vi "Write ITX.vi"(6 "Commands":string, 8 "error in":errorcluster, 9 "Notes":string, 10 "Data (Dictionary)":T1[](array[typedef]), 11 "filename":path) -> (0 "error out":errorcluster, 3 "file":path)   [LabVIEW 2019, in "LV-Data.ITX.lvclass"]
uses:
  LV-Data.ITX.lvclass
  LV-Data/Typedefs/Dictionary--cluster.ctl
  LV-Data/LV-Data.lvclass
panel:
  out "String":string
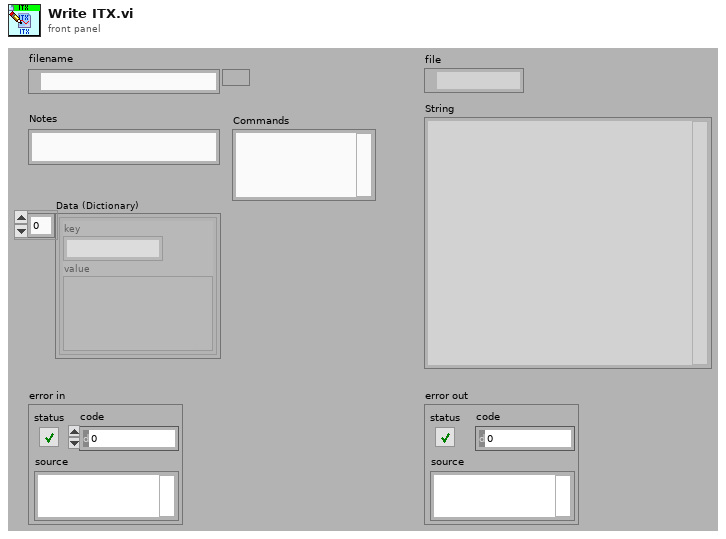
[diagram p1: front panel]
types:
  T1 = typedef "LV-Data.lvclass/Dictionary--cluster.ctl" = cluster{"key":string, "value":variant}
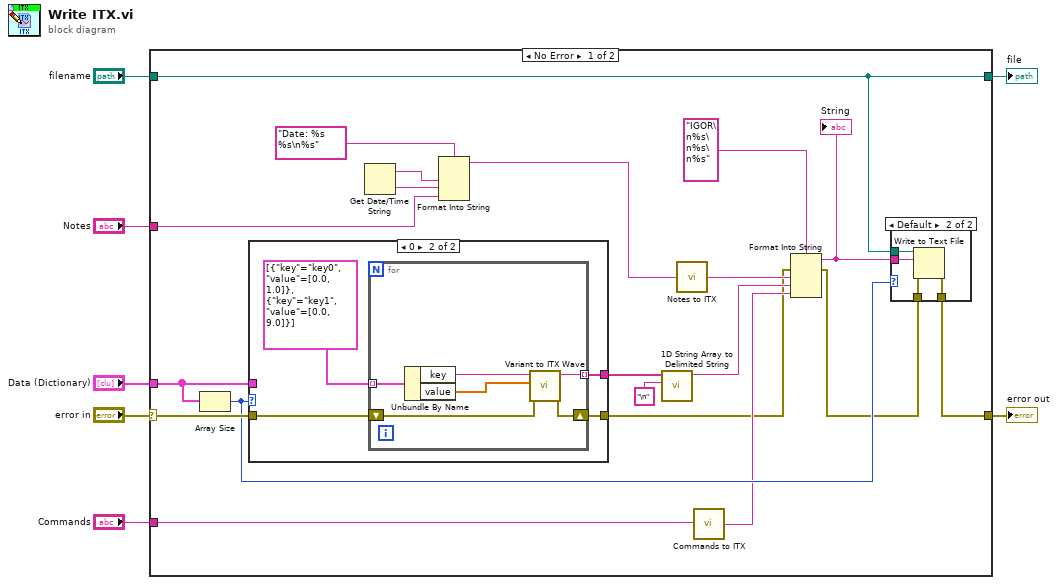
[diagram p0: block diagram]
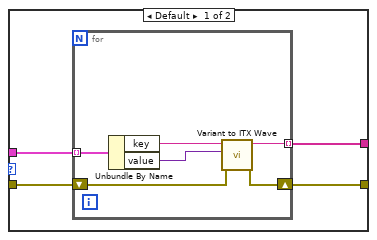
[diagram p2: hidden frame]
diagram:
  n1 = case shown="No Error" "error in" {
    selector: "error in" -> [w24 w53]
    tunnel: "filename" -> [w25 w54]
    tunnel: "Notes" -> [w9 _]
    tunnel: [w27 w53] -> w5
    tunnel: "Data (Dictionary)" -> [w26 _]
    tunnel: [w25 w54] -> w3
    tunnel: "Commands" -> [w23 _]
    frame No Error {
      n2 = Array Size(array=w26) -> (size(s)=w21:i32)
      n3 = case shown="0" w21 {
        tunnel: [w31 w41] -> w22
        tunnel: w26 -> [w30 _]
        tunnel: w24 -> [w29 w40]
        tunnel: [w28 w39] -> w16
        frame Default {
          n4 = for {
            tunnel: [w34] -> w31 mode=indexing
            tunnel: w30 -> [w37] mode=indexing
            shift-right: [w32] -> w28
            shift-left: w29 -> [w33]
            n5 = Unbundle By Name(w37) -> ("key"=w35:string, "value"=w36:variant)
            n6 = call "Variant to ITX Wave.vi"("error in (no error)"=w33, "2D Array"=w36, "Wavename"=w35) -> ("error out"=w32:errorcluster, "ITX Wave"=w34:string)  [unwired: 7 in]
          }
        }
        frame 0 {
          n7 = for {
            tunnel: [w44] -> w41 mode=indexing
            tunnel: cluster{"key":string, "value":dbl[]}[] [{"key"="key0", "value"=[0.0, 1.0]}, {"key"="key1", "value"=[0.0, 9.0]}] ("Data (Dictionary)") -> [w47] mode=indexing
            shift-right: [w43] -> w39
            shift-left: w40 -> [w42]
            n8 = Unbundle By Name(w47) -> ("key"=w45:string, "value"=w46:dbl[])
            n9 = call "Variant to ITX Wave.vi"("error in (no error)"=w42, "2D Array"=w46, "Wavename"=w45) -> ("error out"=w43:errorcluster, "ITX Wave"=w44:string)  [unwired: 7 in]
          }
        }
      }
      n10 = Get Date/Time String() -> (date string=w11:string, time string=w12:string)  [unwired: 3 out]
      n11 = Format Into String(format string="Date: %s %s\n%s", w11, w12, w9) -> (resulting string=w8:string)  [unwired: 2 in, 1 out]
      n12 = call <vilib>:"1D String Array to Delimited String.vi"("delimiter"="\n" ("delimiter (Tab)"), "string array"=w22) -> ("delimited string"=w19:string)  [unwired: 9 in]
      n13 = call "Notes to ITX.vi"("Notes"=w8) -> ("ITX Notes"=w20:string)
      n14 = call "Commands to ITX.vi"("Commands"=w23) -> ("ITX Commands"=w18:string)
      n15 = Format Into String(format string="IGOR\n%s\n%s\n%s", error in=w16, w20, w19, w18) -> (resulting string=w14:string, error out=w15:errorcluster)  [unwired: 1 in]
      "String" <- w14
      n16 = case shown="Default" w21 {
        tunnel: w14 -> [_ w52]
        tunnel: [w48 w51] -> w27
        tunnel: w15 -> [w48 w50]
        tunnel: w25 -> [_ w49]
        frame 0 {
        }
        frame Default {
          n17 = Write to Text File(file (use dialog)=w49, text=w52, error in=w50) -> (error out=w51:errorcluster)  [unwired: 3 out]
        }
      }
    }
    frame Error {
    }
  }
  "file" <- w3
  "error out" <- w5
